vi "Control Mode Select.vi"(8 "Control Mode Read":u16[](array[numeric]), 9 "Power Read":dbl[](array[numeric]), 10 "Voltage Read":dbl[](array[numeric]), 11 "Current Read":dbl[](array[numeric])) -> (1 "Power Write":dbl[](array[numeric]), 2 "Voltage Write":dbl[](array[numeric]), 3 "Current Write":dbl[](array[numeric]))   [LabVIEW 2023]
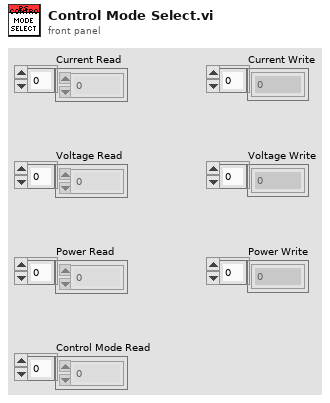
[diagram p1: front panel]
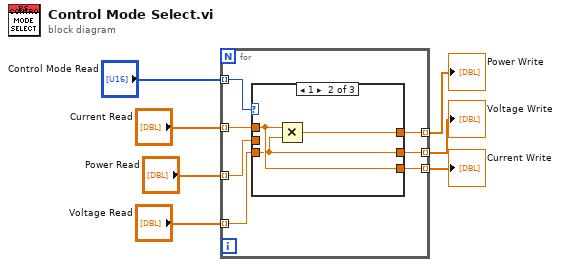
[diagram p0: block diagram]
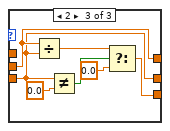
[diagram p3: hidden frame]
diagram:
  n1 = for {
    tunnel: "Control Mode Read" -> [w14] mode=indexing
    tunnel: "Current Read" -> [w13] mode=indexing
    tunnel: [w12] -> w7 mode=indexing
    tunnel: "Voltage Read" -> [w11] mode=indexing
    tunnel: [w10] -> w6 mode=indexing
    tunnel: "Power Read" -> [w9] mode=indexing
    tunnel: [w8] -> w5 mode=indexing
    n2 = case shown="1" w14 {
      tunnel: w13 -> [w17 w20 _]
      tunnel: [w17 w20 w21] -> w12
      tunnel: w11 -> [w16 w19 w23]
      tunnel: [w16 w19 w23] -> w10
      tunnel: [w15 w18 w24] -> w8
      tunnel: w9 -> [w15 _ w24]
      frame 0, Default {
      }
      frame 1 {
        n3 = Multiply(x=w20, y=w19) -> (x*y=w18:dbl)
      }
      frame 2 {
        n4 = Divide(x=w24, y=w23) -> (x/y=w25:dbl)
        n5 = Not Equal?(x=w23, y=0.0) -> (x != y?=w26:bool)
        n6 = Select(t=w25, s=w26, f=0.0) -> (s? t:f=w21:dbl)
      }
    }
  }
  "Current Write" <- w7
  "Voltage Write" <- w6
  "Power Write" <- w5
